vi "FYP_LabviewGlobal(SubVI).vi"() -> ()   [LabVIEW 2013]
panel:
  out "CurrentQnName":string
  out "Question Order":string="0"
  in  "Answer":string
  out "Get Paper Admin":string
  out "Get Topic Admin":string
  out "Get Theme Admin":string
  out "NoOfQnRunning":dbl=15.0
  in  "Why(Text)":string
  in  "Question":string
  in  "Why":bool
  in  "Precontrol":bool
  out "RanFilenames":string[](array[string])
  out "Get Login Time":string
  out "Get Paper":string
  out "Get Topic":string
  out "Get Theme":string
  in  "Password":string
  in  "Admin no":string
  in  "UserName":string
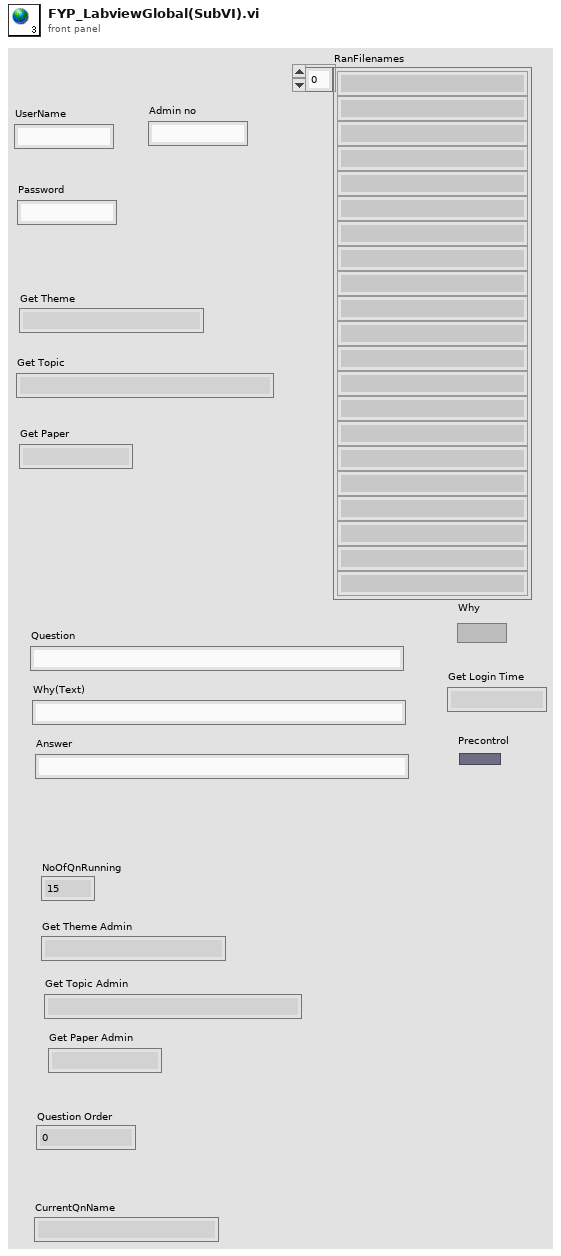
[diagram p1: front panel]
diagram:
